vi "read IO variable U16.vi"(8 "error in (no error)":errorcluster, 9 "data type":u16, 10 "Index":i32=4, 11 "IO Variable Array In":refnum<k21>[](array[refnum])) -> (0 "error out":errorcluster, 2 "data out":u16, 3 "IO Variable Array out":refnum<k21>[](array[refnum]))   [LabVIEW 2016, in "Scan Engine Custom Device.lvlib" / "DS402.lvlib"]
uses:
  DS402.lvlib
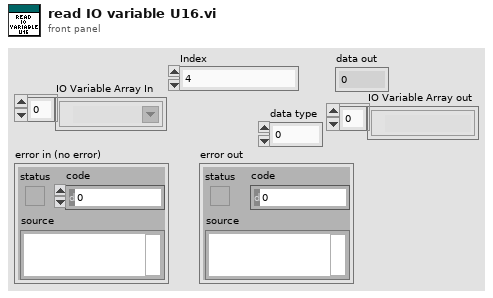
[diagram p1: front panel]
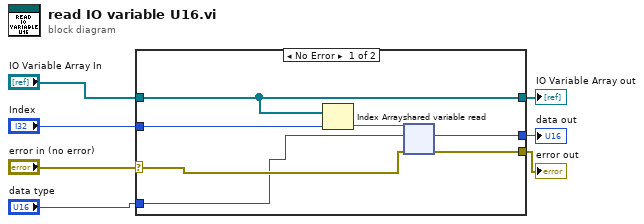
[diagram p0: block diagram]
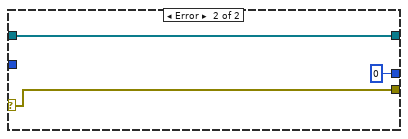
[diagram p2: hidden frame]
diagram:
  n1 = case shown="No Error" "error in (no error)" {
    selector: "error in (no error)" -> [w13 w17]
    tunnel: [w12 w17] -> w6
    tunnel: "IO Variable Array In" -> [w8 w16]
    tunnel: "Index" -> [w11 _]
    tunnel: "data type" -> [w10 _]
    tunnel: [w9 u16 0 ("data type")] -> w2
    tunnel: [w8 w16] -> w1
    frame No Error {
      n2 = Index Array(array=w8, index=w11) -> (element=w14:refnum<k21>)
      n3 = shared-variable-read(w14, w13, w10) -> (w12:errorcluster, w9:u16)  [unwired: 2 out]
    }
    frame Error {
    }
  }
  "error out" <- w6
  "data out" <- w2
  "IO Variable Array out" <- w1
